vi "Source Voltage.vi"(7 "Channel Lists":string[](array[string]), 8 "error in (no error)":errorcluster, 10 "voltage level":dbl format="%_6p", 11 "Instrument Sessions In":refnum<k15>[](array[refnum])) -> (0 "error out":errorcluster, 1 "current measurements":dbl[][](array[numeric]), 2 "voltage measurements":dbl[][](array[numeric]), 3 "Instrument Sessions Out":refnum<k15>[](array[refnum]))   [LabVIEW 2013]
uses:
  <instrlib>/niDCPower/nidcpower.llb/niDCPower Wait For Event - Event.ctl
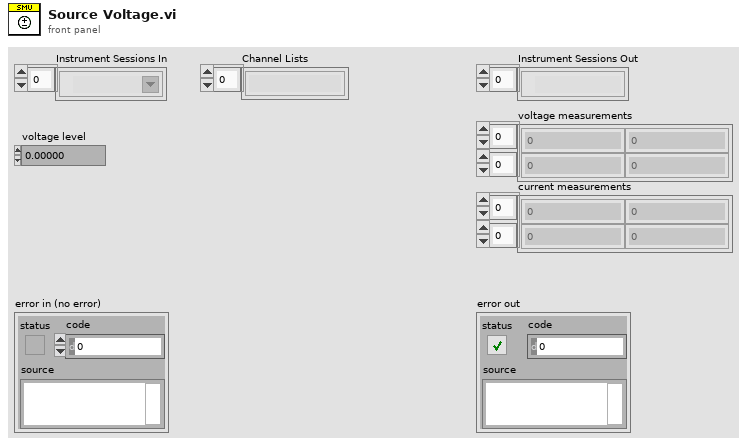
[diagram p1: front panel]
types:
  T1 = typedef "niDCPower Wait For Event - Event.ctl" = i32
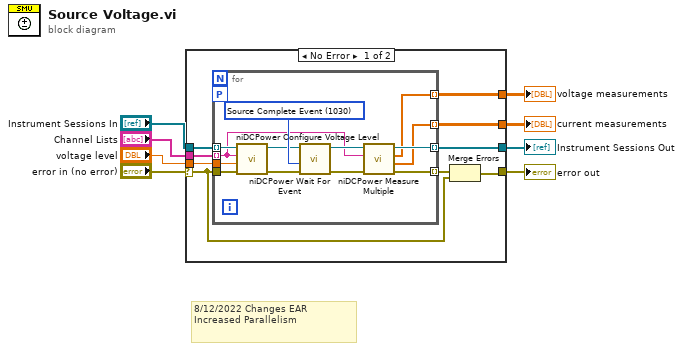
[diagram p0: block diagram]
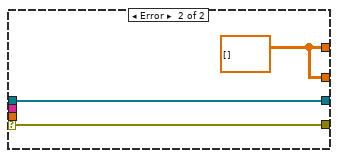
[diagram p2: hidden frame]
diagram:
  # "8/12/2022 Changes EAR\nIncreased Parallelism"
  n1 = case shown="No Error" "error in (no error)" {
    selector: "error in (no error)" -> [w9 w32]
    tunnel: [w16 w32] -> w8
    tunnel: "Instrument Sessions In" -> [w15 w33]
    tunnel: "Channel Lists" -> [w14 _]
    tunnel: [w13 w33] -> w5
    tunnel: "voltage level" -> [w12 _]
    tunnel: [w11 w31] -> w2
    tunnel: [w10 w31] -> w1
    frame No Error {
      n2 = for {
        tunnel: w15 -> [w30] mode=indexing
        tunnel: w14 -> [w22] mode=indexing
        tunnel: [w21] -> w13 mode=indexing
        tunnel: [w20] -> w17 mode=indexing
        tunnel: w12 -> [w29]
        tunnel: w9 -> [w28]
        tunnel: [w19] -> w11 mode=indexing
        tunnel: [w18] -> w10 mode=indexing
        workers-P: _ -> [_]
        w26 = T1 1030 items=["Source Complete Event"=1030, "Measure Complete Event"=1031, "Sequence Iteration Complete Event"=1032, "Sequence Engine Done Event"=1033, "Pulse Complete Event"=1051, "Ready For Pulse Trigger Event"=1052] ("event")
        n3 = call <instrlib>:"niDCPower Configure Voltage Level.vi"("error in (no error)"=w28, "voltage level"=w29, "channel name"=w22, "instrument handle"=w30) -> ("error out"=w27:errorcluster, "instrument handle out"=w25:refnum<k15>)  [unwired: 6 in]
        n4 = call <instrlib>:"niDCPower Wait For Event.vi"("error in (no error)"=w27, "event"=w26, "instrument handle"=w25) -> ("error out"=w24:errorcluster, "instrument handle out"=w23:refnum<k15>)  [unwired: 7 in]
        n5 = call <instrlib>:"niDCPower Measure Multiple.vi"("error in (no error)"=w24, "channel name"=w22, "instrument handle"=w23) -> ("error out"=w20:errorcluster, "current measurements"=w18:dbl[], "voltage measurements"=w19:dbl[], "instrument handle out"=w21:refnum<k15>)  [unwired: 5 in]
      }
      n6 = Merge Errors(w17, w9) -> (w16:errorcluster)
    }
    frame Error {
      w31 = dbl[][] [] ("voltage measurements")
    }
  }
  "Instrument Sessions Out" <- w5
  "error out" <- w8
  "voltage measurements" <- w2
  "current measurements" <- w1
